vi "数字量输入配置.vi"() -> ()   [LabVIEW 2010] (continued)
                        n8012 = Index Array(array=w255, index (row) #1=0 ("索引"), index (row) #2=1 ("索引"), index (row) #3=2 ("索引"), index (row) #4=3 ("索引"), index (row) #5=4 ("索引"), index (row) #6=5 ("索引"), index (row) #7=6 ("索引"), index (row) #8=7 ("索引"), index (row) #9=8 ("索引"), index (row) #10=9 ("索引"), index (row) #11=10 ("索引"), index (row) #12=11 ("索引"), index (row) #13=12 ("索引"), index (row) #14=13 ("索引"), index (row) #15=14 ("索引"), index (row) #16=15 ("索引")) -> (element #1=w275:cluster{u32, u32}[], element #2=w274:cluster{u32, u32}[], element #3=w273:cluster{u32, u32}[], element #4=w272:cluster{u32, u32}[], element #5=w271:cluster{u32, u32}[], element #6=w260:cluster{u32, u32}[], element #7=w261:cluster{u32, u32}[], element #8=w262:cluster{u32, u32}[], element #9=w263:cluster{u32, u32}[], element #10=w264:cluster{u32, u32}[], element #11=w265:cluster{u32, u32}[], element #12=w266:cluster{u32, u32}[], element #13=w267:cluster{u32, u32}[], element #14=w268:cluster{u32, u32}[], element #15=w269:cluster{u32, u32}[], element #16=w270:cluster{u32, u32}[])  [unwired: 16 in]
                        n8013 = local write "D_IN_1"(w256) -> ()
                        n8014 = property on="light_1" class="Bool (严格)"("Colors [4]"=w275) -> ()  [unwired: 2 in, 2 out]
                        n8015 = property on="light_2" class="Bool (严格)"("Colors [4]"=w274) -> ()  [unwired: 2 in, 2 out]
                        n8016 = property on="light_3" class="Bool (严格)"("Colors [4]"=w273) -> ()  [unwired: 2 in, 2 out]
                        n8017 = property on="light_4" class="Bool (严格)"("Colors [4]"=w272) -> ()  [unwired: 2 in, 2 out]
                        n8018 = property on="light_5" class="Bool (严格)"("Colors [4]"=w271) -> ()  [unwired: 2 in, 2 out]
                        n8019 = property on="light_6" class="Bool (严格)"("Colors [4]"=w260) -> ()  [unwired: 2 in, 2 out]
                        n8020 = property on="light_7" class="Bool (严格)"("Colors [4]"=w261) -> ()  [unwired: 2 in, 2 out]
                        n8021 = property on="light_8" class="Bool (严格)"("Colors [4]"=w262) -> ()  [unwired: 2 in, 2 out]
                        n8022 = property on="light_9" class="Bool (严格)"("Colors [4]"=w263) -> ()  [unwired: 2 in, 2 out]
                        n8023 = property on="light_10" class="Bool (严格)"("Colors [4]"=w264) -> ()  [unwired: 2 in, 2 out]
                        n8024 = property on="light_11" class="Bool (严格)"("Colors [4]"=w265) -> ()  [unwired: 2 in, 2 out]
                        n8025 = property on="light_12" class="Bool (严格)"("Colors [4]"=w266) -> ()  [unwired: 2 in, 2 out]
                        n8026 = property on="light_13" class="Bool (严格)"("Colors [4]"=w267) -> ()  [unwired: 2 in, 2 out]
                        n8027 = property on="light_14" class="Bool (严格)"("Colors [4]"=w268) -> ()  [unwired: 2 in, 2 out]
                        n8028 = property on="light_15" class="Bool (严格)"("Colors [4]"=w269) -> ()  [unwired: 2 in, 2 out]
                        n8029 = property on="light_16" class="Bool (严格)"("Colors [4]"=w270) -> ()  [unwired: 2 in, 2 out]
                      }
                      frame 2 {
                        n8030 = local read "D_IN_3"() -> (w294:string[][])
                        n8031 = Replace Array Subset(array=w294, new element=w293, index (col)=2 ("索引 (列)")) -> (w292:string[][])  [unwired: 1 in]
                        n8032 = Index Array(array=w312, index (row) #1=0 ("索引"), index (row) #2=1 ("索引"), index (row) #3=2 ("索引"), index (row) #4=3 ("索引"), index (row) #5=4 ("索引"), index (row) #6=5 ("索引"), index (row) #7=6 ("索引"), index (row) #8=7 ("索引"), index (row) #9=8 ("索引"), index (row) #10=9 ("索引"), index (row) #11=10 ("索引"), index (row) #12=11 ("索引"), index (row) #13=12 ("索引"), index (row) #14=13 ("索引"), index (row) #15=14 ("索引"), index (row) #16=15 ("索引")) -> (element #1=w311:cluster{u32, u32}[], element #2=w310:cluster{u32, u32}[], element #3=w309:cluster{u32, u32}[], element #4=w308:cluster{u32, u32}[], element #5=w307:cluster{u32, u32}[], element #6=w306:cluster{u32, u32}[], element #7=w305:cluster{u32, u32}[], element #8=w304:cluster{u32, u32}[], element #9=w303:cluster{u32, u32}[], element #10=w302:cluster{u32, u32}[], element #11=w301:cluster{u32, u32}[], element #12=w300:cluster{u32, u32}[], element #13=w299:cluster{u32, u32}[], element #14=w298:cluster{u32, u32}[], element #15=w297:cluster{u32, u32}[], element #16=w296:cluster{u32, u32}[])  [unwired: 16 in]
                        n8033 = local write "D_IN_3"(w292) -> ()
                        n8034 = property on="light_33" class="Bool (严格)"("Colors [4]"=w311) -> ()  [unwired: 2 in, 2 out]
                        n8035 = property on="light_34" class="Bool (严格)"("Colors [4]"=w310) -> ()  [unwired: 2 in, 2 out]
                        n8036 = property on="light_35" class="Bool (严格)"("Colors [4]"=w309) -> ()  [unwired: 2 in, 2 out]
                        n8037 = property on="light_36" class="Bool (严格)"("Colors [4]"=w308) -> ()  [unwired: 2 in, 2 out]
                        n8038 = property on="light_37" class="Bool (严格)"("Colors [4]"=w307) -> ()  [unwired: 2 in, 2 out]
                        n8039 = property on="light_38" class="Bool (严格)"("Colors [4]"=w306) -> ()  [unwired: 2 in, 2 out]
                        n8040 = property on="light_39" class="Bool (严格)"("Colors [4]"=w305) -> ()  [unwired: 2 in, 2 out]
                        n8041 = property on="light_40" class="Bool (严格)"("Colors [4]"=w304) -> ()  [unwired: 2 in, 2 out]
                        n8042 = property on="light_41" class="Bool (严格)"("Colors [4]"=w303) -> ()  [unwired: 2 in, 2 out]
                        n8043 = property on="light_42" class="Bool (严格)"("Colors [4]"=w302) -> ()  [unwired: 2 in, 2 out]
                        n8044 = property on="light_43" class="Bool (严格)"("Colors [4]"=w301) -> ()  [unwired: 2 in, 2 out]
                        n8045 = property on="light_44" class="Bool (严格)"("Colors [4]"=w300) -> ()  [unwired: 2 in, 2 out]
                        n8046 = property on="light_45" class="Bool (严格)"("Colors [4]"=w299) -> ()  [unwired: 2 in, 2 out]
                        n8047 = property on="light_46" class="Bool (严格)"("Colors [4]"=w298) -> ()  [unwired: 2 in, 2 out]
                        n8048 = property on="light_47" class="Bool (严格)"("Colors [4]"=w297) -> ()  [unwired: 2 in, 2 out]
                        n8049 = property on="light_48" class="Bool (严格)"("Colors [4]"=w296) -> ()  [unwired: 2 in, 2 out]
                      }
                      frame 3 {
                        n8050 = local read "D_IN_4"() -> (w331:string[][])
                        n8051 = Replace Array Subset(array=w331, new element=w330, index (col)=2 ("索引 (列)")) -> (w329:string[][])  [unwired: 1 in]
                        n8052 = Index Array(array=w349, index (row) #1=0 ("索引"), index (row) #2=1 ("索引"), index (row) #3=2 ("索引"), index (row) #4=3 ("索引"), index (row) #5=4 ("索引"), index (row) #6=5 ("索引"), index (row) #7=6 ("索引"), index (row) #8=7 ("索引"), index (row) #9=8 ("索引"), index (row) #10=9 ("索引"), index (row) #11=10 ("索引"), index (row) #12=11 ("索引"), index (row) #13=12 ("索引"), index (row) #14=13 ("索引"), index (row) #15=14 ("索引"), index (row) #16=15 ("索引")) -> (element #1=w348:cluster{u32, u32}[], element #2=w347:cluster{u32, u32}[], element #3=w346:cluster{u32, u32}[], element #4=w345:cluster{u32, u32}[], element #5=w344:cluster{u32, u32}[], element #6=w343:cluster{u32, u32}[], element #7=w342:cluster{u32, u32}[], element #8=w341:cluster{u32, u32}[], element #9=w340:cluster{u32, u32}[], element #10=w339:cluster{u32, u32}[], element #11=w338:cluster{u32, u32}[], element #12=w337:cluster{u32, u32}[], element #13=w336:cluster{u32, u32}[], element #14=w335:cluster{u32, u32}[], element #15=w334:cluster{u32, u32}[], element #16=w333:cluster{u32, u32}[])  [unwired: 16 in]
                        n8053 = local write "D_IN_4"(w329) -> ()
                        n8054 = property on="light_49" class="Bool (严格)"("Colors [4]"=w348) -> ()  [unwired: 2 in, 2 out]
                        n8055 = property on="light_50" class="Bool (严格)"("Colors [4]"=w347) -> ()  [unwired: 2 in, 2 out]
                        n8056 = property on="light_51" class="Bool (严格)"("Colors [4]"=w346) -> ()  [unwired: 2 in, 2 out]
                        n8057 = property on="light_52" class="Bool (严格)"("Colors [4]"=w345) -> ()  [unwired: 2 in, 2 out]
                        n8058 = property on="light_53" class="Bool (严格)"("Colors [4]"=w344) -> ()  [unwired: 2 in, 2 out]
                        n8059 = property on="light_54" class="Bool (严格)"("Colors [4]"=w343) -> ()  [unwired: 2 in, 2 out]
                        n8060 = property on="light_55" class="Bool (严格)"("Colors [4]"=w342) -> ()  [unwired: 2 in, 2 out]
                        n8061 = property on="light_56" class="Bool (严格)"("Colors [4]"=w341) -> ()  [unwired: 2 in, 2 out]
                        n8062 = property on="light_57" class="Bool (严格)"("Colors [4]"=w340) -> ()  [unwired: 2 in, 2 out]
                        n8063 = property on="light_58" class="Bool (严格)"("Colors [4]"=w339) -> ()  [unwired: 2 in, 2 out]
                        n8064 = property on="light_59" class="Bool (严格)"("Colors [4]"=w338) -> ()  [unwired: 2 in, 2 out]
                        n8065 = property on="light_60" class="Bool (严格)"("Colors [4]"=w337) -> ()  [unwired: 2 in, 2 out]
                        n8066 = property on="light_61" class="Bool (严格)"("Colors [4]"=w336) -> ()  [unwired: 2 in, 2 out]
                        n8067 = property on="light_62" class="Bool (严格)"("Colors [4]"=w335) -> ()  [unwired: 2 in, 2 out]
                        n8068 = property on="light_63" class="Bool (严格)"("Colors [4]"=w334) -> ()  [unwired: 2 in, 2 out]
                        n8069 = property on="light_64" class="Bool (严格)"("Colors [4]"=w333) -> ()  [unwired: 2 in, 2 out]
                      }
                      frame 4 {
                        n8070 = local read "D_IN_5"() -> (w368:string[][])
                        n8071 = Replace Array Subset(array=w368, new element=w366, index (col)=2 ("索引 (列)")) -> (w367:string[][])  [unwired: 1 in]
                        n8072 = Index Array(array=w386, index (row) #1=0 ("索引"), index (row) #2=1 ("索引"), index (row) #3=2 ("索引"), index (row) #4=3 ("索引"), index (row) #5=4 ("索引"), index (row) #6=5 ("索引"), index (row) #7=6 ("索引"), index (row) #8=7 ("索引"), index (row) #9=8 ("索引"), index (row) #10=9 ("索引"), index (row) #11=10 ("索引"), index (row) #12=11 ("索引"), index (row) #13=12 ("索引"), index (row) #14=13 ("索引"), index (row) #15=14 ("索引"), index (row) #16=15 ("索引")) -> (element #1=w385:cluster{u32, u32}[], element #2=w384:cluster{u32, u32}[], element #3=w383:cluster{u32, u32}[], element #4=w382:cluster{u32, u32}[], element #5=w381:cluster{u32, u32}[], element #6=w380:cluster{u32, u32}[], element #7=w379:cluster{u32, u32}[], element #8=w378:cluster{u32, u32}[], element #9=w377:cluster{u32, u32}[], element #10=w376:cluster{u32, u32}[], element #11=w375:cluster{u32, u32}[], element #12=w374:cluster{u32, u32}[], element #13=w373:cluster{u32, u32}[], element #14=w372:cluster{u32, u32}[], element #15=w371:cluster{u32, u32}[], element #16=w370:cluster{u32, u32}[])  [unwired: 16 in]
                        n8073 = local write "D_IN_5"(w367) -> ()
                        n8074 = property on="light_65" class="Bool (严格)"("Colors [4]"=w385) -> ()  [unwired: 2 in, 2 out]
                        n8075 = property on="light_66" class="Bool (严格)"("Colors [4]"=w384) -> ()  [unwired: 2 in, 2 out]
                        n8076 = property on="light_67" class="Bool (严格)"("Colors [4]"=w383) -> ()  [unwired: 2 in, 2 out]
                        n8077 = property on="light_68" class="Bool (严格)"("Colors [4]"=w382) -> ()  [unwired: 2 in, 2 out]
                        n8078 = property on="light_69" class="Bool (严格)"("Colors [4]"=w381) -> ()  [unwired: 2 in, 2 out]
                        n8079 = property on="light_70" class="Bool (严格)"("Colors [4]"=w380) -> ()  [unwired: 2 in, 2 out]
                        n8080 = property on="light_71" class="Bool (严格)"("Colors [4]"=w379) -> ()  [unwired: 2 in, 2 out]
                        n8081 = property on="light_72" class="Bool (严格)"("Colors [4]"=w378) -> ()  [unwired: 2 in, 2 out]
                        n8082 = property on="light_73" class="Bool (严格)"("Colors [4]"=w377) -> ()  [unwired: 2 in, 2 out]
                        n8083 = property on="light_74" class="Bool (严格)"("Colors [4]"=w376) -> ()  [unwired: 2 in, 2 out]
                        n8084 = property on="light_75" class="Bool (严格)"("Colors [4]"=w375) -> ()  [unwired: 2 in, 2 out]
                        n8085 = property on="light_76" class="Bool (严格)"("Colors [4]"=w374) -> ()  [unwired: 2 in, 2 out]
                        n8086 = property on="light_77" class="Bool (严格)"("Colors [4]"=w373) -> ()  [unwired: 2 in, 2 out]
                        n8087 = property on="light_78" class="Bool (严格)"("Colors [4]"=w372) -> ()  [unwired: 2 in, 2 out]
                        n8088 = property on="light_79" class="Bool (严格)"("Colors [4]"=w371) -> ()  [unwired: 2 in, 2 out]
                        n8089 = property on="light_80" class="Bool (严格)"("Colors [4]"=w370) -> ()  [unwired: 2 in, 2 out]
                      }
                      frame 1 {
                        n8090 = local read "D_IN_2"() -> (w405:string[][])
                        n8091 = Replace Array Subset(array=w405, new element=w403, index (col)=2 ("索引 (列)")) -> (w404:string[][])  [unwired: 1 in]
                        n8092 = Index Array(array=w423, index (row) #1=0 ("索引"), index (row) #2=1 ("索引"), index (row) #3=2 ("索引"), index (row) #4=3 ("索引"), index (row) #5=4 ("索引"), index (row) #6=5 ("索引"), index (row) #7=6 ("索引"), index (row) #8=7 ("索引"), index (row) #9=8 ("索引"), index (row) #10=9 ("索引"), index (row) #11=10 ("索引"), index (row) #12=11 ("索引"), index (row) #13=12 ("索引"), index (row) #14=13 ("索引"), index (row) #15=14 ("索引"), index (row) #16=15 ("索引")) -> (element #1=w422:cluster{u32, u32}[], element #2=w421:cluster{u32, u32}[], element #3=w420:cluster{u32, u32}[], element #4=w419:cluster{u32, u32}[], element #5=w418:cluster{u32, u32}[], element #6=w417:cluster{u32, u32}[], element #7=w416:cluster{u32, u32}[], element #8=w415:cluster{u32, u32}[], element #9=w414:cluster{u32, u32}[], element #10=w413:cluster{u32, u32}[], element #11=w412:cluster{u32, u32}[], element #12=w411:cluster{u32, u32}[], element #13=w410:cluster{u32, u32}[], element #14=w409:cluster{u32, u32}[], element #15=w408:cluster{u32, u32}[], element #16=w407:cluster{u32, u32}[])  [unwired: 16 in]
                        n8093 = local write "D_IN_2"(w404) -> ()
                        n8094 = property on="light_17" class="Bool (严格)"("Colors [4]"=w422) -> ()  [unwired: 2 in, 2 out]
                        n8095 = property on="light_18" class="Bool (严格)"("Colors [4]"=w421) -> ()  [unwired: 2 in, 2 out]
                        n8096 = property on="light_19" class="Bool (严格)"("Colors [4]"=w420) -> ()  [unwired: 2 in, 2 out]
                        n8097 = property on="light_20" class="Bool (严格)"("Colors [4]"=w419) -> ()  [unwired: 2 in, 2 out]
                        n8098 = property on="light_21" class="Bool (严格)"("Colors [4]"=w418) -> ()  [unwired: 2 in, 2 out]
                        n8099 = property on="light_22" class="Bool (严格)"("Colors [4]"=w417) -> ()  [unwired: 2 in, 2 out]
                        n8100 = property on="light_23" class="Bool (严格)"("Colors [4]"=w416) -> ()  [unwired: 2 in, 2 out]
                        n8101 = property on="light_24" class="Bool (严格)"("Colors [4]"=w415) -> ()  [unwired: 2 in, 2 out]
                        n8102 = property on="light_25" class="Bool (严格)"("Colors [4]"=w414) -> ()  [unwired: 2 in, 2 out]
                        n8103 = property on="light_26" class="Bool (严格)"("Colors [4]"=w413) -> ()  [unwired: 2 in, 2 out]
                        n8104 = property on="light_27" class="Bool (严格)"("Colors [4]"=w412) -> ()  [unwired: 2 in, 2 out]
                        n8105 = property on="light_28" class="Bool (严格)"("Colors [4]"=w411) -> ()  [unwired: 2 in, 2 out]
                        n8106 = property on="light_29" class="Bool (严格)"("Colors [4]"=w410) -> ()  [unwired: 2 in, 2 out]
                        n8107 = property on="light_30" class="Bool (严格)"("Colors [4]"=w409) -> ()  [unwired: 2 in, 2 out]
                        n8108 = property on="light_31" class="Bool (严格)"("Colors [4]"=w408) -> ()  [unwired: 2 in, 2 out]
                        n8109 = property on="light_32" class="Bool (严格)"("Colors [4]"=w407) -> ()  [unwired: 2 in, 2 out]
                      }
                    }
                    n8110 = local read "测试结论"() -> (w245:string)
                    n8111 = case shown="真" w248 {
                      tunnel: [w445 w451] -> w252
                      tunnel: w245 -> [w446 w452]
                      tunnel: w237 -> [w441 w449]
                      frame False {
                        n8112 = Increment(x=w441) -> (x+1=w440:i32)
                        n8113 = Format Into String(format string="被测板卡第%d路数字量输入测试故障，\n具体见上面试验结论！", w440) -> (resulting string=w443:string)  [unwired: 2 in, 1 out]
                        n8114 = Concatenate Strings(w446, w443, "\r") -> (w445:string)
                      }
                      frame True {
                        n8115 = Format Into String(format string="被测板卡第%d路数字量输入正常！", w449) -> (resulting string=w448:string)  [unwired: 2 in, 1 out]
                        n8116 = Concatenate Strings(w452, w448, "\r") -> (w451:string)
                      }
                    }
                    n8117 = local write "测试结论"(w252) -> ()
                  }
                }
              }
              frame #1 {
                n8118 = local read "保持输入"() -> (w453:bool)
                n8119 = case shown="假" w453 {
                  frame False {
                    n8120 = local read "同步_A2"() -> (w455:i32)
                    n8121 = Increment(x=w455) -> (x+1=w454:i32)
                    n8122 = local write "同步_A2"(w454) -> ()
                  }
                  frame True {
                  }
                }
              }
            }
          }
        }
        n8123 = local read "关闭？"() -> (w216:bool)
      }
      n8124 = Release Notifier(notifier=w201, error in (no error)=w200) -> ()  [unwired: 1 in, 3 out]
    }
  }
  n8125 = disable-structure shown="禁用" {
    frame Disabled {
      n8126 = for {
        N: 40 -> [_]
        i -> [w1017]
        n8127 = for {
          N: 4 -> [_]
          tunnel: w1017 -> [w1025]
          i -> [w1022]
          n8128 = Bundle(w1025, w1022) -> (w1021:cluster{i32, i32})  [unwired: 1 in]
          n8129 = Quotient & Remainder(x=w1025, y=2) -> (x-y*floor(x/y)=w1023:i32)  [unwired: 1 out]
          n8130 = property on="D_IN_1" class="Tbl (严格)"("Active Cell"=w1021) -> (error out=w1019:errorcluster)  [unwired: 2 in, 1 out]
          n8131 = Equal To 0?(x=w1023) -> (x = 0?=w1026:bool)
          n8132 = case shown="真" w1026 {
            tunnel: [u32 16448250 u32 15723488] -> w1020
            frame False {
            }
            frame True {
            }
          }
          n8133 = property on="D_IN_1" class="Tbl (严格)"(error in=w1019, "Cell BG Color"=w1020) -> ()  [unwired: 1 in, 2 out]
        }
        n8134 = Wait Until Next ms Multiple(millisecond multiple=u32 10 ("毫秒倍数")) -> ()  [unwired: 1 out]
      }
    }
    frame Enabled {
    }
  }
  n8135 = disable-structure shown="禁用" {
    frame Disabled {
      n8136 = for {
        N: 40 -> [_]
        i -> [w1034]
        n8137 = Wait Until Next ms Multiple(millisecond multiple=u32 10 ("毫秒倍数")) -> ()  [unwired: 1 out]
        n8138 = Bundle(w1034, "y"=-1) -> (w1033:cluster{i32, "y":i32})  [unwired: 1 in]
        n8139 = property on="D_IN_1" class="Tbl (严格)"("Active Cell"=w1033) -> (error out=w1032:errorcluster)  [unwired: 2 in, 1 out]
        n8140 = property on="D_IN_1" class="Tbl (严格)"(error in=w1032, "Cell BG Color"=u32 12369084) -> ()  [unwired: 1 in, 2 out]
      }
    }
    frame Enabled {
    }
  }
